vi "Parse-element.vi"(8 "error in (no error)":errorcluster, 10 "String in":string, 11 "WriteAnalog in":refnum<class "WriteAnalog.lvclass">) -> (0 "error out":errorcluster, 1 "Valid element?":bool, 2 "Remaining string":string, 3 "WriteAnalog out":refnum<class "WriteAnalog.lvclass">)   [LabVIEW 2013, in "HardwareCharacterization.lvlib" / "WriteAnalog.lvclass"]
uses:
  WriteAnalog.lvclass
  WriteAnalog.lvclass/WriteAnalog.ctl
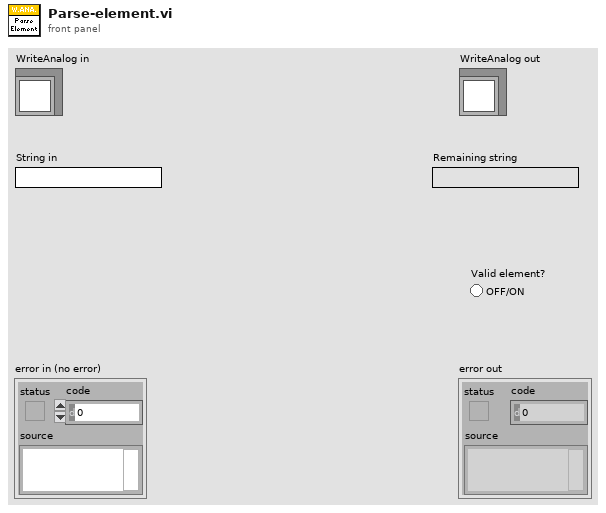
[diagram p1: front panel]
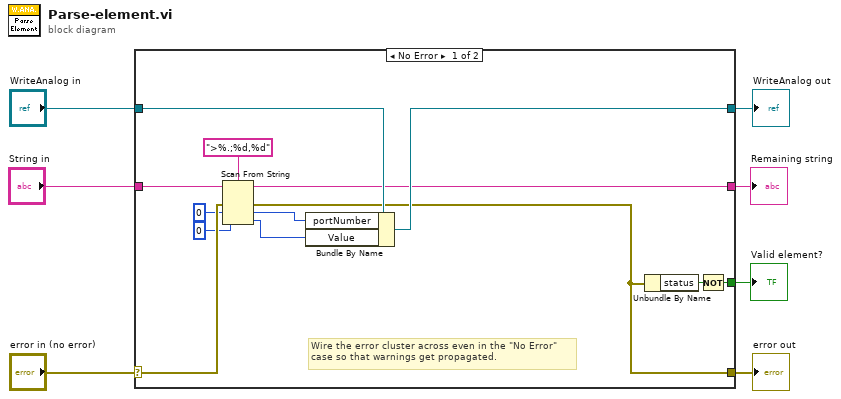
[diagram p0: block diagram]
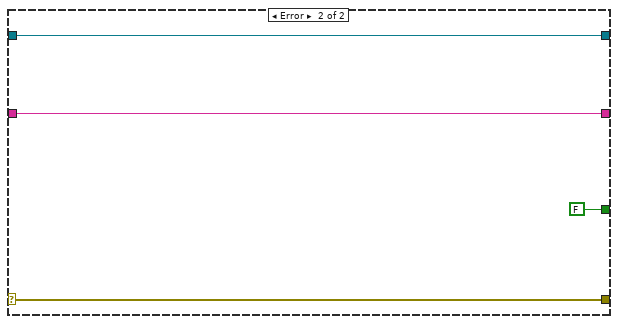
[diagram p2: hidden frame]
diagram:
  n1 = case shown="No Error" "error in (no error)" {
    selector: "error in (no error)" -> [w15 w24]
    tunnel: [w8 w24] -> w6
    tunnel: [w11 w23] -> w4
    tunnel: "WriteAnalog in" -> [w12 w23]
    tunnel: "String in" -> [w16 w22]
    tunnel: [w10 w22] -> w2
    tunnel: [w9 FALSE] -> w1
    frame No Error {
      # "Wire the error cluster across even in the \"No Error\"\ncase so that warnings get propagated."
      n2 = Scan From String(format string=">%.;%d,%d", input string=w16, error in=w15, default 1=u8 0 ("default value 2"), default 2=u16 0 ("default value 3")) -> (remaining string=w10:string, error out=w8:errorcluster, output 1=w18:u8, output 2=w17:u16)  [unwired: 1 in, 1 out]
      n3 = Bundle By Name(cluster=w12, "portNumber"=w18, "Value"=w17) -> (w11:refnum<class "WriteAnalog.lvclass">)
      n4 = Unbundle By Name(w8) -> ("status"=w19:bool)
      n5 = Not(x=w19) -> (.not. x?=w9:bool)
    }
    frame Error {
    }
  }
  "error out" <- w6
  "WriteAnalog out" <- w4
  "Remaining string" <- w2
  "Valid element?" <- w1
